vi "Climb Control Loop.vi"() -> ()   [LabVIEW 2019]
uses:
  Calculations or utilities/Is command done typedef.ctl
  <vilib>/Rock Robotics/WPI/ThirdParty/Phoenix-LabVIEW/Motor Controller/Controls/CTRE_Phoenix_MotorControl_ControlMode.ctl
  Climb Global.vi
  <vilib>/Rock Robotics/WPI/ThirdParty/Phoenix-LabVIEW/Motor Controller/Get/CTRE_Phoenix_MotorController_GetLimitSwitchStates.vi
panel:
  out "Reverse Limit Closed?":bool
  out "Forward Limit Closed?":bool
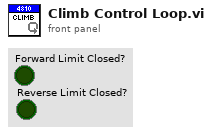
[diagram p1: front panel]
types:
  T1 = typedef "WPI_MotorControlDeviceRef.ctl" = cluster{"DeviceStatus":errorcluster, "Type":T2, "PWM":cluster{"PWM Channel":T3, "DeadBand":T4}, "CAN":cluster{"Device Number":u8, "SetOutput VI Ref":variant, "GetOutput VI Ref":variant, "Enable VI Ref":variant, "Disable VI Ref":variant, "Data":variant}, "Invert":bool, "DIO PWM":cluster{"PWM \"Enable\" Channel":T3, "DIOChannel":T5, "PWM Rate":dbl}}
  T2 = typedef "WPI_MotorControlType.ctl" = enum16{"PWM", "CAN", "DIO PWM"}
  T3 = typedef "FPGA_DIOPWMChannel.ctl" = enum8{"PWM 0", "PWM 1", "PWM 2", "PWM 3", "PWM 4", "PWM 5", "PWM 6", "PWM 7", "PWM 8", "PWM 9", "PWM MXP 0", "PWM MXP 1", "PWM MXP 2", "PWM MXP 3", "PWM MXP 4", "PWM MXP 5", "PWM MXP 6", "PWM MXP 7", "PWM MXP 8", "PWM MXP 9", "Invalid"}
  T4 = typedef "WPI_PWMDeadband.ctl" = cluster{"Name":string, "maxPositivePwm":i32, "minPositivePwm":i32, "centerPwm":i32, "maxNegativePwm":i32, "minNegativePwm":i32, "angularRange":u16}
  T5 = typedef "FPGA_DIOChannel.ctl" = enum8{"DIO 0", "DIO 1", "DIO 2", "DIO 3", "DIO 4", "DIO 5", "DIO 6", "DIO 7", "DIO 8", "DIO 9", "DIO MXP 0", "DIO MXP 1", "DIO MXP 2", "DIO MXP 3", "DIO MXP 4", "DIO MXP 5", "DIO MXP 6", "DIO MXP 7", "DIO MXP 8", "DIO MXP 9", "DIO MXP 10", "DIO MXP 11", "DIO MXP 12", "DIO MXP 13", "DIO MXP 14", "DIO MXP 15", "SPI Port CS1", "SPI Port CS2", "SPI Port CS3", "SPI Port MISO", "SPI Port MOSI", "Invalid"}
  T6 = typedef "Is command done typedef.ctl" = cluster{"Done?":bool, "Timestamp [ms]":dbl}
  T7 = typedef "Climb Command Type Def.ctl" = cluster{"Climb Mode":T8, "Throttle (%)":dbl, "Timestamp (ms)":dbl, "Skywalker Throttle (%)":dbl}
  T8 = typedef "Climb Mode Type Def.ctl" = enum16{"Disabled", "Raw Throttle"}
  T9 = typedef "CTRE_Phoenix_MotorControl_ControlMode.ctl" = u16
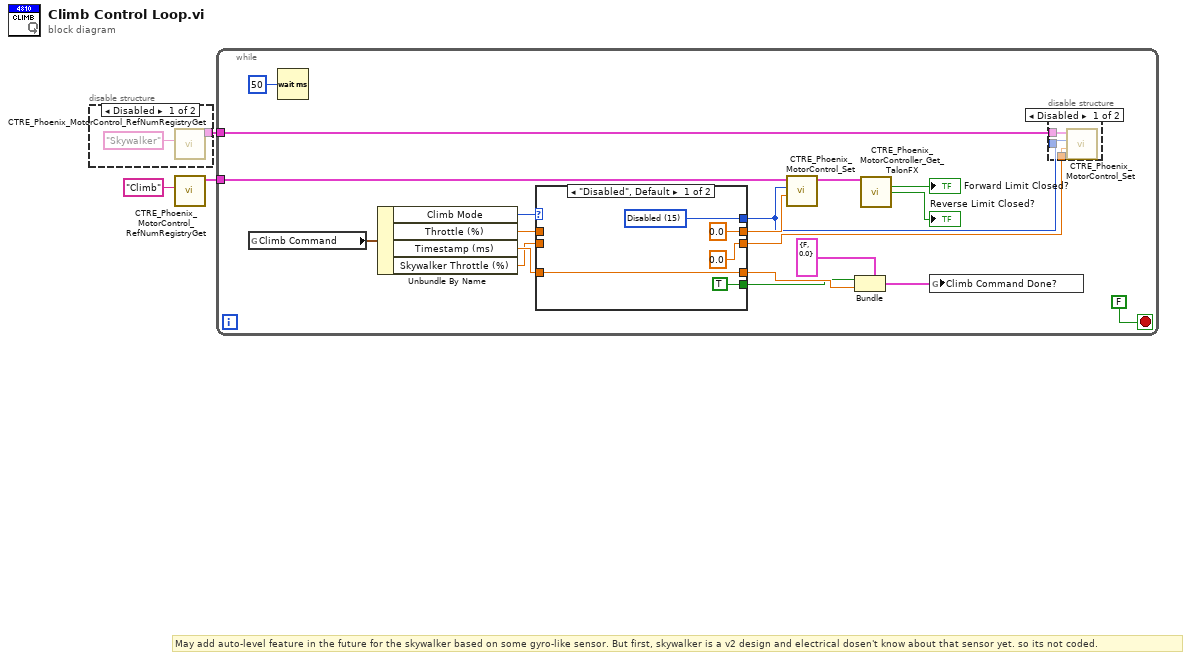
[diagram p0: block diagram]
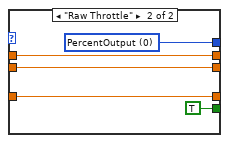
[diagram p4: hidden frame]
diagram:
  # "May add auto-level feature in the future for the skywalker based on some gyro-like sensor. But first, skywalker is a v2 design and electrical dosen't know about that sensor yet. so its not coded."
  n1 = disable-structure shown="Disabled" {
    disable-tunnel: [w4 _] -> w1
    frame Disabled {
      n2 = call <vilib>:"CTRE_Phoenix_MotorControl_RefNumRegistryGet.vi"("refnum name"="Skywalker") -> ("PhoenixMotorControlDevRef"=w4:T1)  [unwired: 9 in, 1 out]
    }
    frame Enabled {
    }
  }
  n3 = call <vilib>:"CTRE_Phoenix_MotorControl_RefNumRegistryGet.vi"("refnum name"="Climb") -> ("PhoenixMotorControlDevRef"=w2:T1)  [unwired: 9 in, 1 out]
  n4 = while {
    tunnel: w2 -> [w22]
    tunnel: w1 -> [w12]
    stop <- FALSE stop-if-true
    n5 = global read "Climb Global.vi" "Climb Command"() -> (w13:T7)
    n6 = Wait (ms)(milliseconds to wait=u32 50) -> ()  [unwired: 1 out]
    n7 = Unbundle By Name(w13) -> ("Climb Mode"=w21:T8, "Throttle (%)"=w18:dbl, "Timestamp (ms)"=w20:dbl, "Skywalker Throttle (%)"=w8:dbl)
    n8 = case shown="\"Disabled\", Default" w21 {
      tunnel: [w32 w35] -> w6
      tunnel: [w31 w36] -> w16
      tunnel: w20 -> [w31 w36]
      tunnel: [0.0 ("Throttle (%)") w37] -> w19
      tunnel: w18 -> [_ w37]
      tunnel: [TRUE ("Done?") TRUE ("Done?")] -> w15
      tunnel: w8 -> [_ w33]
      tunnel: [0.0 ("Skywalker Throttle (%)") w33] -> w7
      frame "Disabled", Default {
        w32 = T9 15 items=["PercentOutput"=0, "Position"=1, "Velocity"=2, "Current"=3, "Follower"=5, "MotionProfile"=6, "MotionMagic"=7, "MotionProfileArc"=10, "Disabled"=15] ("Control Mode")
      }
      frame "Raw Throttle" {
        w35 = T9 0 items=["PercentOutput"=0, "Position"=1, "Velocity"=2, "Current"=3, "Follower"=5, "MotionProfile"=6, "MotionMagic"=7, "MotionProfileArc"=10, "Disabled"=15] ("Control Mode")
      }
    }
    n9 = call <vilib>:"CTRE_Phoenix_MotorControl_Set.vi"("Output"=w19, "Control Mode"=w6, "PhoenixMotorControlDevRef"=w22) -> ("PhoenixMotorControlDevRef"=w11:T1)  [unwired: 7 in, 1 out]
    n10 = Bundle(cluster=T6 {"Done?"=FALSE, "Timestamp [ms]"=0.0} ("Command Done?"), "Done?"=w15, "Timestamp [ms]"=w16) -> (w14:T6)
    n11 = call-poly <vilib>:"CTRE_Phoenix_MotorController_Get_TalonFX.vi"("PhoenixMotorControlDevRef"=w11) -> ("Forward Limit Closed?"=→"Forward Limit Closed?":bool, "Reverse Limit Closed?"=→"Reverse Limit Closed?":bool)  [unwired: 11 in, 2 out]
    n12 = global write "Climb Global.vi" "Climb Command Done?"(w14) -> ()
    n13 = disable-structure shown="Disabled" {
      disable-tunnel: w12 -> [w27 _]
      disable-tunnel: w7 -> [w26 _]
      disable-tunnel: w6 -> [w25 _]
      frame Disabled {
        n14 = call <vilib>:"CTRE_Phoenix_MotorControl_Set.vi"("Output"=w26, "Control Mode"=w25, "PhoenixMotorControlDevRef"=w27) -> ()  [unwired: 7 in, 2 out]
      }
      frame Enabled {
      }
    }
  }
